vi "Calculate Power Spectrum (1D CDB WDT).vi"(0 "IQ Waveforms":waveform(cdb)[](array[waveform])) -> (4 "power spectra":cluster{"f0":dbl, "df":dbl, "magnitude":dbl[]}[](array[cluster]))   [LabVIEW 2015]
doc: "Calculates the power spectrum from the I/Q waveform."
uses:
  <vilib>/measure/maspectr.llb/FFT Power Spectrum and PSD for 1 Chan (CDB).vi
  <vilib>/measure/NI_MAPro.lvlib
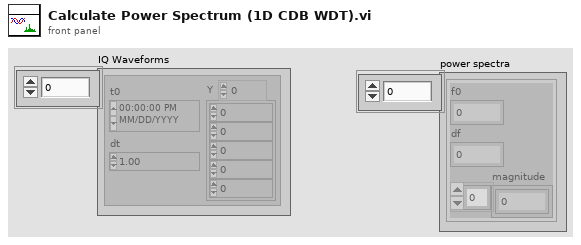
[diagram p1: front panel]
types:
  T1 = cluster{"averaging mode":enum16{"No averaging", "Vector averaging", "RMS averaging", "Peak hold"}, "weighting mode":enum16{"Linear", "Exponential"}, "number of averages":u32}
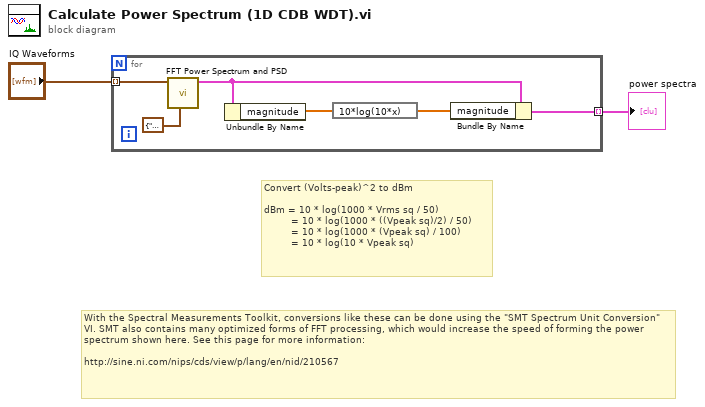
[diagram p0: block diagram]
diagram:
  # "With the Spectral Measurements Toolkit, conversions like these can be done using the \"SMT Spectrum Unit Conversion\" VI. SMT also contains many optimized forms of FFT processing, which would increase the speed of forming the power spectrum shown here. See this page for more information: \n\nhttp://sine.ni.com/nips/cds/view/p/lang/en/nid/210567"
  # "Convert (Volts-peak)^2 to dBm\n\ndBm = 10 * log(1000 * Vrms sq / 50)\n         = 10 * log(1000 * ((Vpeak sq)/2) / 50) \n         = 10 * log(1000 * (Vpeak sq) / 100) \n         = 10 * log(10 * Vpeak sq)"
  n1 = for {
    tunnel: "IQ Waveforms" -> [w4] mode=indexing
    tunnel: [w3] -> w1 mode=indexing
    n2 = call-poly <vilib>:"FFT Power Spectrum and PSD.vi"("averaging parameters"=T1 {"averaging mode"=enum."No averaging", "weighting mode"=enum."Exponential", "number of averages"=10}, "time signal"=w4) -> ("Power Spectrum / PSD"=w6:cluster{"f0":dbl, "df":dbl, "magnitude":dbl[]})  [unwired: 6 in, 3 out]
    n3 = Unbundle By Name(w6) -> ("magnitude"=w7:dbl[])
    n4 = expression code="10*log(10*x)"(w7) -> (w8:dbl[])
    n5 = Bundle By Name(cluster=w6, "magnitude"=w8) -> (w3:cluster{"f0":dbl, "df":dbl, "magnitude":dbl[]})
  }
  "power spectra" <- w1
